vi "Read Session Information.vi"(8 "error in (no error)":errorcluster, 11 "TwinCAT ADS in":refnum<class "TwinCAT ADS.lvclass">) -> (0 "error out":errorcluster, 1 "Session Infomation":T1 {"Capabilities" items=["None"=0, "DataTypeSupport"=1, "SymbolBrowsing"=2, "ValueRead"=4, "ValueWrite"=8, "ValueNotifications"=16, "Mask_All"=31]; "Connection State" items=["None, Unknown", "Disconnected", "Connected", "Lost"]}, 3 "TwinCAT ADS out":refnum<class "TwinCAT ADS.lvclass">)   [LabVIEW 2018, in "TwinCAT ADS.lvclass"]
uses:
  TwinCAT ADS.lvclass
  Controls/Session Information.ctl
  TwinCAT ADS.lvclass/TwinCAT ADS.ctl
  TwinCAT.Ads
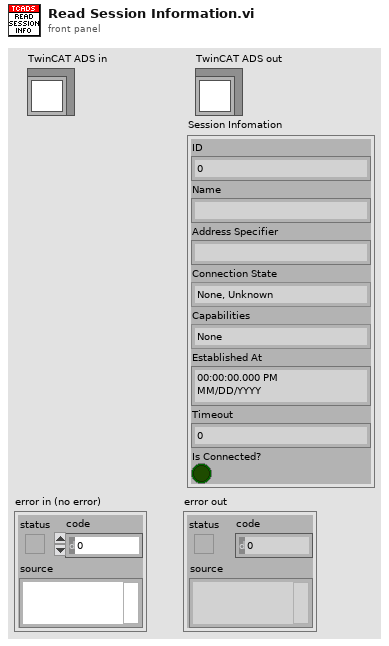
[diagram p1: front panel]
types:
  T1 = typedef "TwinCAT ADS.lvclass/Session Information.ctl" = cluster{"ID":i32, "Name":string, "Address Specifier":string, "Connection State":i32, "Capabilities":i32, "Established At":timestamp, "Timeout":i32, "Is Connected?":bool}
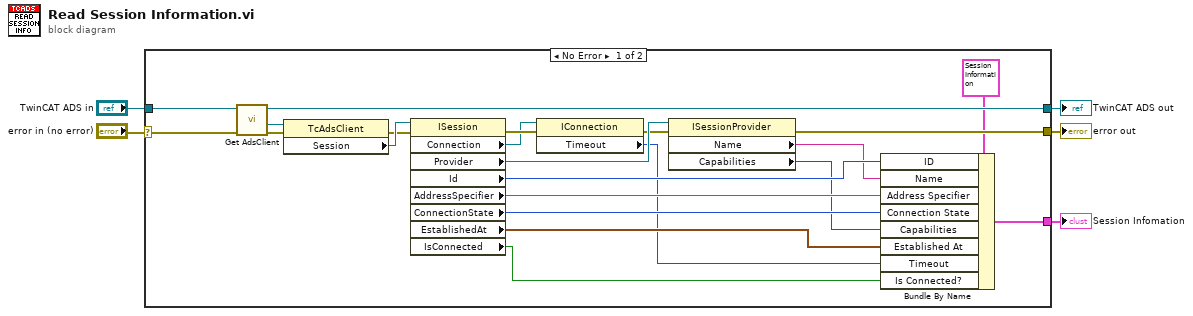
[diagram p0: block diagram]
diagram:
  n1 = case shown="No Error" "error in (no error)" {
    selector: "error in (no error)" -> [w9 w29]
    tunnel: [w14 w29] -> w4
    tunnel: [w7 w28] -> w2
    tunnel: "TwinCAT ADS in" -> [w8 w28]
    tunnel: [w13 _] -> w1
    frame No Error {
      n2 = call "Get AdsClient.vi"("error in (no error)"=w9, "TwinCAT ADS in"=w8) -> ("error out"=w11:errorcluster, ".NET TcAdsClient refnum"=w10:refnum<k24>, "TwinCAT ADS out"=w7:refnum<class "TwinCAT ADS.lvclass">)  [unwired: 7 in]
      n3 = property class="TcAdsClient"(reference=w10, error in=w11) -> (error out=w26:errorcluster, "Session"=w27:refnum<k24>)  [unwired: 1 out]
      n4 = property class="ISession"(reference=w27, error in=w26) -> (error out=w25:errorcluster, "Connection"=w12:refnum<k24>, "Provider"=w24:refnum<k24>, "Id"=w22:i32, "AddressSpecifier"=w20:string, "ConnectionState"=w19:i32, "EstablishedAt"=w17:timestamp, "IsConnected"=w15:bool)  [unwired: 1 out]
      n5 = property class="IConnection"(reference=w12, error in=w25) -> (error out=w23:errorcluster, "Timeout"=w16:i32)  [unwired: 1 out]
      n6 = property class="ISessionProvider"(reference=w24, error in=w23) -> (error out=w14:errorcluster, "Name"=w21:string, "Capabilities"=w18:i32)  [unwired: 1 out]
      n7 = Bundle By Name(cluster=T1 {"ID"=0, "Name"="", "Address Specifier"="", "Connection State"=0, "Capabilities"=0, "Established At"=timestamp(0 s since 1904-01-01), "Timeout"=0, "Is Connected?"=FALSE} ("Session Infomation"), "ID"=w22, "Name"=w21, "Address Specifier"=w20, "Connection State"=w19, "Capabilities"=w18, "Established At"=w17, "Timeout"=w16, "Is Connected?"=w15) -> (w13:T1)
    }
    frame Error {
    }
  }
  "error out" <- w4
  "TwinCAT ADS out" <- w2
  "Session Infomation" <- w1
